vi "farbanpassung einzug.vi"(8 "error in (no error)":errorcluster caption="Fehler (Eingang, kein Fehler)", 11 "Device ID":T1(ring)) -> (0 "error out":errorcluster caption="Fehler (Ausgang)")   [LabVIEW 2010]
panel:
  out "Numerisches Element":i32
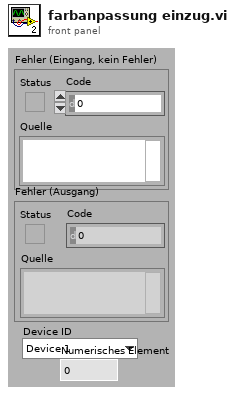
[diagram p1: front panel]
types:
  T1 = enum16{"Device 1", "Device 2", "Device 3", "Device 4", "Device 5", "Device 6", "Device 7", "Device 8"}
  T2 = enum8{"Power 1", "Power 2", "Power 3", "Power 4", "Power 5", "Power 6", "Power 7", "Power 8"}
  T3 = enum8{"Output 1 (O1)", "Output 2 (O2)", "Output 3 (O3)", "Output 4 (O4)", "Output 5 (O5)", "Output 6 (O6)", "Output 7 (O7)", "Output 8 (O8)"}
  T4 = enum8{"Robo Interface", "Extension 1", "Extension 2", "Extension 3"}
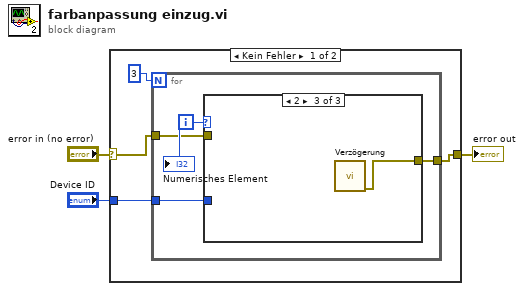
[diagram p0: block diagram]
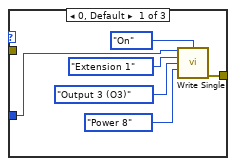
[diagram p2: hidden frame]
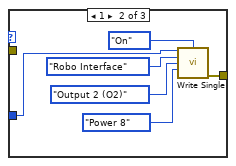
[diagram p3: hidden frame]
diagram:
  n1 = case shown="Kein Fehler" "error in (no error)" {
    selector: "error in (no error)" -> [w4 w25]
    tunnel: [w5 w25] -> w2
    tunnel: "Device ID" -> [w6 _]
    frame No Error {
      n2 = for {
        N: 3 -> [_]
        tunnel: w6 -> [w10]
        tunnel: [w9] -> w5
        tunnel: w4 -> [w8]
        i -> [w11]
        n3 = case shown="2" w11 {
          tunnel: w10 -> [w17 w22 _]
          tunnel: [w12 w23 w24] -> w9
          tunnel: w8 -> [_ _ _]
          frame 0, Default {
            n4 = call "Write Single.vi"("Device ID"=w17, "Output_Action"=enum8{"Off", "On"}."On", "Module"=T4."Extension 1", "Single_Output"=T3."Output 3 (O3)", "Output_PWM"=T2."Power 8") -> ("error out"=w12:errorcluster)  [unwired: 1 in, 9 out]
          }
          frame 1 {
            n5 = call "Write Single.vi"("Device ID"=w22, "Output_Action"=enum8{"Off", "On"}."On", "Module"=T4."Robo Interface", "Single_Output"=T3."Output 2 (O2)", "Output_PWM"=T2."Power 8") -> ("error out"=w23:errorcluster)  [unwired: 1 in, 9 out]
          }
          frame 2 {
            n6 = call "Verzögerung"() -> ("error out"=w24:errorcluster)  [unwired: 2 in, 9 out]
          }
        }
        "Numerisches Element" <- w11
      }
    }
    frame Error {
    }
  }
  "error out" <- w2
